vi "Read_Write ParaINI File1.vi"(5 "Mode":enum16{"Read", "Write"}(ring), 6 "Indicators too?":bool, 7 "Section":string, 8 "error in":errorcluster, 9 "Filepath":path, 11 "Ctl Refnum":refnum<vi>) -> (0 "error out":errorcluster)   [LabVIEW 2019]
uses:
  <vilib>/Utility/config.llb/NI_LVConfig.lvlib
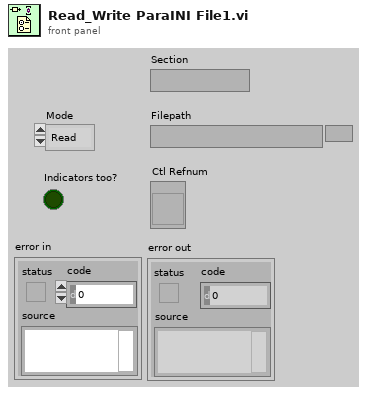
[diagram p1: front panel]
types:
  T1 = typedef "NI_LVConfig.lvlib/Config Data RefNum.ctl" = refnum<k1>
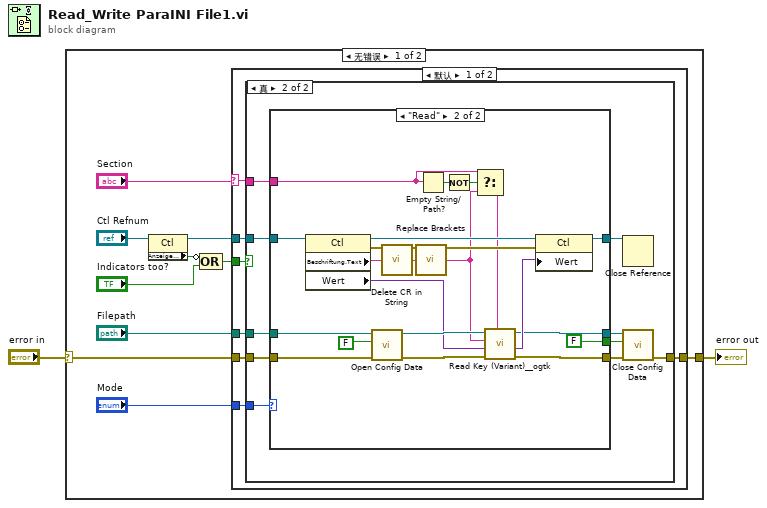
[diagram p0: block diagram]
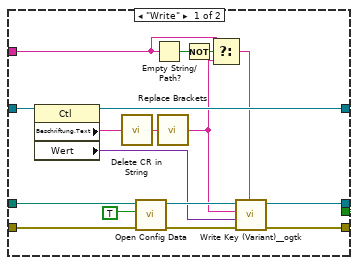
[diagram p3: hidden frame]
diagram:
  n1 = case shown="无错误" "error in" {
    selector: "error in" -> [w9 w71]
    tunnel: [w12 w71] -> w1
    frame No Error {
      n2 = property class="Ctl"(reference="Ctl Refnum") -> (reference out=w8:refnum<vi>, "Anzeigeelement"=w6:bool)  [unwired: 1 in, 1 out]
      n3 = Compound Arithmetic op=OR(invert w6, "Indicators too?") -> (w4:bool)
      n4 = case shown="默认" "Section" {
        selector: "Section" -> [w13 _]
        tunnel: [w19 w70] -> w12
        tunnel: "Mode" -> [w18 _]
        tunnel: "Filepath" -> [w17 _]
        tunnel: w9 -> [w16 w70]
        tunnel: w8 -> [w15 _]
        tunnel: w4 -> [w14 _]
        frame Default {
          n5 = case shown="真" w14 {
            tunnel: w13 -> [_ w30]
            tunnel: [w20 w21] -> w19
            tunnel: w18 -> [_ w29]
            tunnel: w17 -> [_ w28]
            tunnel: w16 -> [w20 w27]
            tunnel: w15 -> [_ w25]
            frame False {
            }
            frame True {
              n6 = case shown="\"Read\"" w29 {
                tunnel: [w32 w55] -> w22
                tunnel: [w33 w62] -> w24
                tunnel: w30 -> [w38 w50]
                tunnel: w27 -> [w45 w65]
                tunnel: w25 -> [w48 w69]
                tunnel: [TRUE ("write configuration file? (F)") FALSE ("write configuration file? (F)")] -> w23
                tunnel: w28 -> [w44 w67]
                tunnel: [w42 w63] -> w26
                frame "Write" {
                  n7 = property class="Ctl"(reference=w48) -> (reference out=w42:refnum<vi>, "Beschriftung.Text"=w41:string, "Wert"=w36:variant)  [unwired: 1 in, 1 out]
                  n8 = call "Delete CR in String.vi"("Input String"=w41) -> ("String without CR"=w43:string)  [unwired: 4 out]
                  n9 = call <vilib>:"Open Config Data.vi"("error in (no error)"=w45, "create file if necessary (T)"=TRUE ("create file if necessary? (T)"), "configuration file path"=w44) -> ("error out"=w34:errorcluster, "refnum"=w37:T1)  [unwired: 6 in, 1 out]
                  n10 = Empty String/Path?(string/path=w38) -> (empty?=w40:bool)
                  n11 = call "Replace Brackets.vi"("Label.Text"=w43) -> ("String"=w31:string)  [unwired: 4 out]
                  n12 = Not(x=w40) -> (.not. x?=w39:bool)
                  n13 = Select(t=w38, s=w39, f=w31) -> (s? t:f=w35:string)
                  n14 = call "Write Key (Variant)__ogtk.vi"("section"=w35, "error in (no error)"=w34, "key-value"=w36, "key (optional)"=w31, "refnum"=w37) -> ("error out"=w33:errorcluster, "refnum out"=w32:T1)  [unwired: 5 in]
                }
                frame "Read" {
                  n15 = property class="Ctl"(reference=w69) -> (reference out=w56:refnum<vi>, error out=w57:errorcluster, "Beschriftung.Text"=w54:string, "Wert"=w58:variant)  [unwired: 1 in]
                  n16 = call <vilib>:"Open Config Data.vi"("error in (no error)"=w65, "create file if necessary (T)"=FALSE ("create file if necessary? (T)"), "configuration file path"=w67) -> ("error out"=w59:errorcluster, "refnum"=w60:T1)  [unwired: 6 in, 1 out]
                  n17 = call "Delete CR in String.vi"("Input String"=w54) -> ("String without CR"=w64:string)  [unwired: 4 in]
                  n18 = call "Replace Brackets.vi"("Label.Text"=w64) -> ("String"=w49:string)  [unwired: 4 in]
                  n19 = Empty String/Path?(string/path=w50) -> (empty?=w53:bool)
                  n20 = Not(x=w53) -> (.not. x?=w52:bool)
                  n21 = Select(t=w50, s=w52, f=w49) -> (s? t:f=w51:string)
                  n22 = call "Read Key (Variant)__ogtk.vi"("section"=w51, "error in (no error)"=w59, "type"=w58, "key (optional)"=w49, "refnum"=w60) -> ("error out"=w62:errorcluster, "key-value"=w61:variant, "refnum out"=w55:T1)  [unwired: 3 in, 1 out]
                  n23 = property class="Ctl"(reference=w56, error in=w57, "Wert"=w61) -> (reference out=w63:refnum<vi>)  [unwired: 1 out]
                }
              }
              n24 = Close Reference(reference=w26) -> ()  [unwired: 1 in, 1 out]
              n25 = call <vilib>:"Close Config Data.vi"("error in (no error)"=w24, "write file if changed (T)"=w23, "refnum"=w22) -> ("error out"=w21:errorcluster)  [unwired: 7 in, 1 out]
            }
          }
        }
        frame "" {
        }
      }
    }
    frame Error {
    }
  }
  "error out" <- w1
